vi "LAC_H410 example.vi"() -> ()   [LabVIEW 2014]
uses:
  TypeDef/H410 Cmd_exec TypeDef.ctl
panel:
  out "ERR?":bool
  in  "cmd":string="R103,0" caption="cmd (w/o LF CR)"
  in  "VISA resource name":refnum<visa-resource-name>="COM5"
  out "array out":string[](array[string])
  in  "error in":errorcluster
  out "error out":errorcluster
  out "read buffer":string
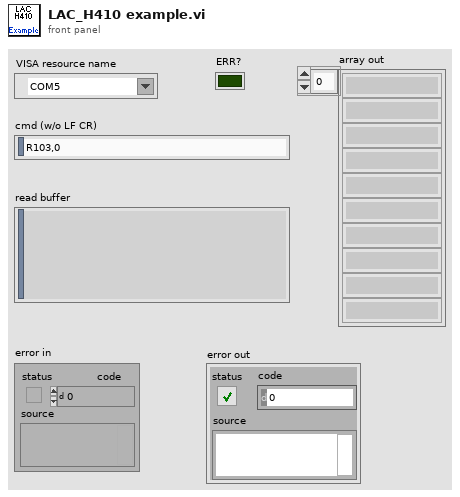
[diagram p1: front panel]
types:
  T1 = typedef "H410 Cmd_exec TypeDef.ctl" = u16
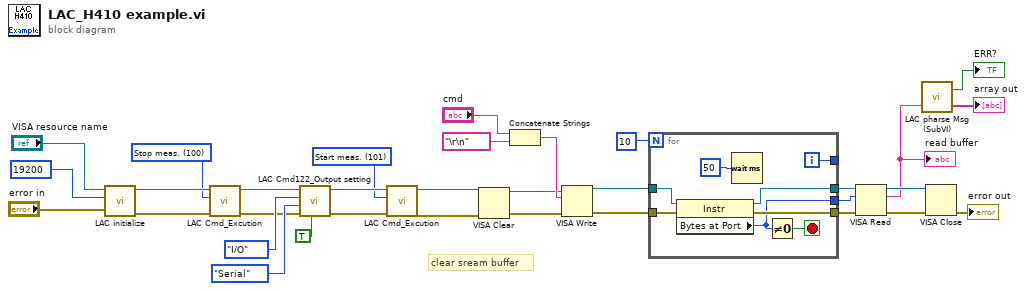
[diagram p0: block diagram]
diagram:
  w16 = T1 100 items=["Stop meas."=100, "Start meas."=101, "Auto-adj. LD output"=105, "Zero reset"=106, "Zero set"=107, "OFFSETTILT judge 1"=108, "OFFSETTILT judge 2"=109] ("Cmd_exec")
  w17 = T1 101 items=["Stop meas."=100, "Start meas."=101, "Auto-adj. LD output"=105, "Zero reset"=106, "Zero set"=107, "OFFSETTILT judge 1"=108, "OFFSETTILT judge 2"=109] ("Cmd_exec")
  # "clear sream buffer"
  n1 = call "LAC initialize.vi"("error in"="error in", "baud rate"=u32 19200 ("baud rate (9600)"), "VISA Refnum in"="VISA resource name") -> ("error out"=w24:errorcluster, "VISA Refnum out"=w25:refnum<visa-resource-name>)  [unwired: 7 in]
  n2 = call "LAC Cmd_Excution.vi"("error in"=w24, "Cmd_exec"=w16, "VISA name in"=w25) -> ("error out"=w18:errorcluster, "VISA name out"=w19:refnum<visa-resource-name>)  [unwired: 6 in, 1 out]
  n3 = call "LAC Cmd122_Output setting.vi"("R/W (F:Read)"=TRUE, "error in"=w18, "Out port"=enum16{"Serial", "Ethernet"}."Serial", "Out mode"=enum16{"Stream", "I/O", "OFF"}."I/O", "VISA name in"=w19) -> ("error out"=w21:errorcluster, "VISA name out"=w20:refnum<visa-resource-name>)  [unwired: 4 in, 1 out]
  n4 = call "LAC Cmd_Excution.vi"("error in"=w21, "Cmd_exec"=w17, "VISA name in"=w20) -> ("error out"=w10:errorcluster, "VISA name out"=w11:refnum<visa-resource-name>)  [unwired: 6 in, 1 out]
  n5 = VISA Clear(VISA resource name=w11, error in (no error)=w10) -> (VISA resource name out=w9:refnum<visa-resource-name>, error out=w8:errorcluster)
  n6 = Concatenate Strings("cmd", "\r\n" ("write buffer")) -> (w13:string)
  n7 = VISA Write(VISA resource name=w9, write buffer=w13, error in (no error)=w8) -> (VISA resource name out=w31:refnum<visa-resource-name>, error out=w30:errorcluster)  [unwired: 1 out]
  n8 = for {
    N: 10 -> [_]
    tunnel: w31 -> [w41]
    tunnel: [w36] -> w7
    tunnel: [w39] -> w5
    tunnel: w30 -> [w38]
    tunnel: [w37] -> w4
    tunnel: [w34] -> _
    i -> [w34]
    stop <- w35 stop-if-true
    n9 = property class="Instr"(reference=w41, error in=w38) -> (reference out=w39:refnum<visa-resource-name>, error out=w37:errorcluster, "Bytes at Port"=w36:u32)
    n10 = Wait (ms)(milliseconds to wait=u32 50) -> ()  [unwired: 1 out]
    n11 = Not Equal To 0?(x=w36) -> (x != 0?=w35:bool)
  }
  n12 = VISA Read(VISA resource name=w5, byte count=w7, error in (no error)=w4) -> (VISA resource name out=w28:refnum<visa-resource-name>, read buffer=w3:string, error out=w29:errorcluster)  [unwired: 1 out]
  "read buffer" <- w3
  n13 = call "LAC pharse Msg (SubVI).vi"("result"=w3) -> ("array out"=→"array out":string[], "ERR?"=→"ERR?":bool)  [unwired: 1 in]
  n14 = VISA Close(VISA resource name=w28, error in (no error)=w29) -> (error out=→"error out":errorcluster)
